vi "全局变量.vi"() -> ()   [LabVIEW 2011]
panel:
  in  "调频（MHz）":dbl
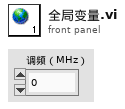
[diagram p1: front panel]
diagram:
